vi "2 Cube Auto.vi"(11 "Right?":bool=TRUE) -> ()   [LabVIEW 2017]
uses:
  Auto Scale Type Def.ctl
  2 Cube Auto Type Def.ctl
  LabVIEW_is_Under_Control.lib/Util/Unpack Gamepad/D-Pad.ctl
  LabVIEW_is_Under_Control.lib/Util/Unpack Gamepad/Button Cluster.ctl
  Team Code/Robot Global Data.vi
panel:
  in  "String":string
  in  "DistanceFwd 4":dbl=600.0
  in  "Delay Fwd 4":i32=300
  in  "Time_Limit_fwd 4":dbl=5000.0 format="%#_13g"
  in  "Time_Limit_Turn 2":dbl=1000.0 format="%#_13g"
  in  "Turn 2":dbl=-30.0 format="%#_13g"
  in  "Delay Turn 2":i32=100
  in  "DistanceFwd 3":dbl=-60.0
  in  "Delay Fwd 3":i32=100
  in  "Time_Limit_fwd 3":dbl=1000.0 format="%#_13g"
  in  "Time to wait 3 (min 50ms)":dbl=100.0
  in  "DistanceFwd 2":dbl=55.0
  in  "Delay Fwd 2":i32=100
  in  "Time_Limit_fwd 2":dbl=1000.0 format="%#_13g"
  in  "Time to wait 2 (min 50ms)":dbl=100.0
  in  "Time_Limit_Turn":dbl=1000.0 format="%#_13g"
  in  "Turn":dbl=-30.0 format="%#_13g"
  in  "Delay Turn":i32=100
  in  "DistanceFwd":dbl=600.0
  in  "Delay Fwd":i32=300
  in  "Time_Limit_fwd":dbl=5000.0 format="%#_13g"
  in  "Time to wait (min 50ms)":dbl=100.0
  out "Auto state":T1=enum."Finalizando"
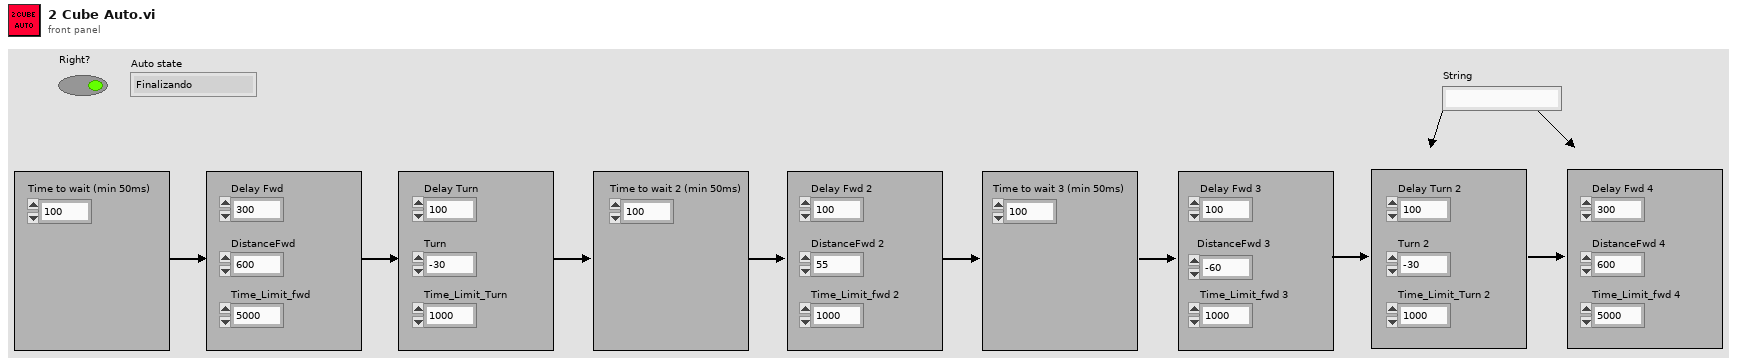
[diagram p1: front panel]
types:
  T1 = typedef "Auto Scale Type Def.ctl" = enum16{"Zerandosensor", "Andando", "Girando", "Zerandosensor2", "Andando2", "Score", "Zerandosensor3", "Andando3", "Finalizando"}
  T2 = typedef "2 Cube Auto Type Def.ctl" = enum16{"Zerandosensor", "Andando", "Girando", "Zerandosensor2", "Andando2", "Score", "Zerandosensor3", "Andando3", "Girando2", "Andando4", "Elevator Up", "Score2", "Finalizando"}
  T3 = typedef "D-Pad.ctl" = cluster{"Top":bool, "Bottom":bool, "None":bool, "Right":bool, "Left":bool}
  T4 = cluster{"proportional gain (Kc)":dbl, "integral time (Ti, min)":dbl, "derivative time (Td, min)":dbl}
  T5 = typedef "Button Cluster.ctl" = cluster{"Buttons[0]":bool, "Buttons[1]":bool, "Buttons[2]":bool, "Buttons[3]":bool, "Buttons[4]":bool, "Buttons[5]":bool, "Buttons[6]":bool, "Buttons[7]":bool, "Buttons[8]":bool, "Buttons[9]":bool}
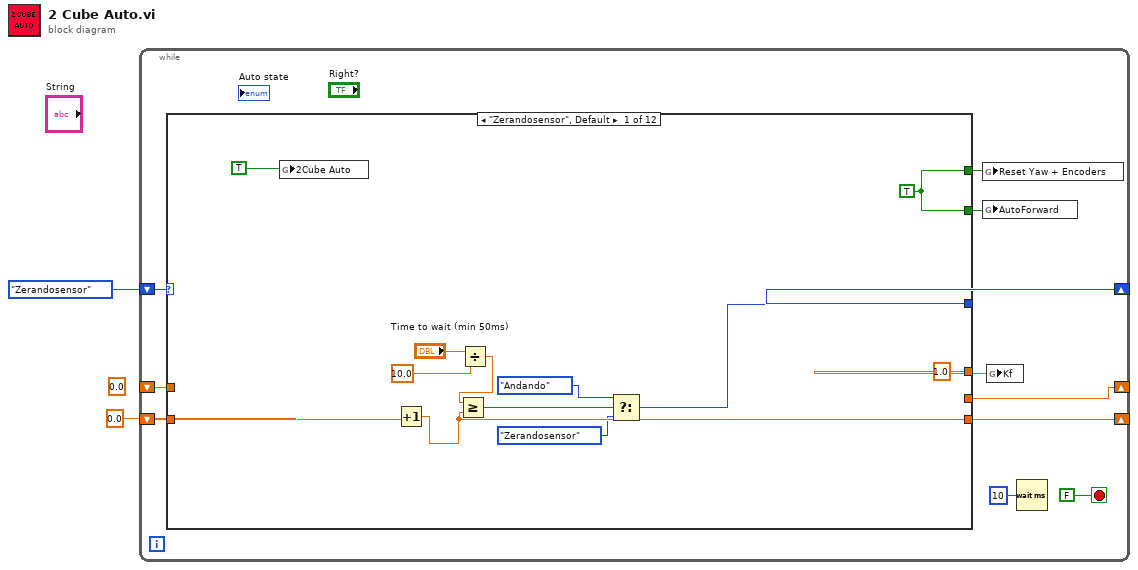
[diagram p0: block diagram]
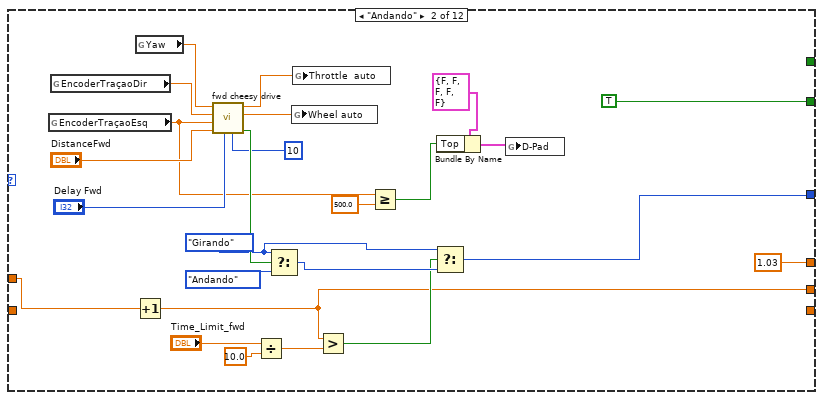
[diagram p2: hidden frame]
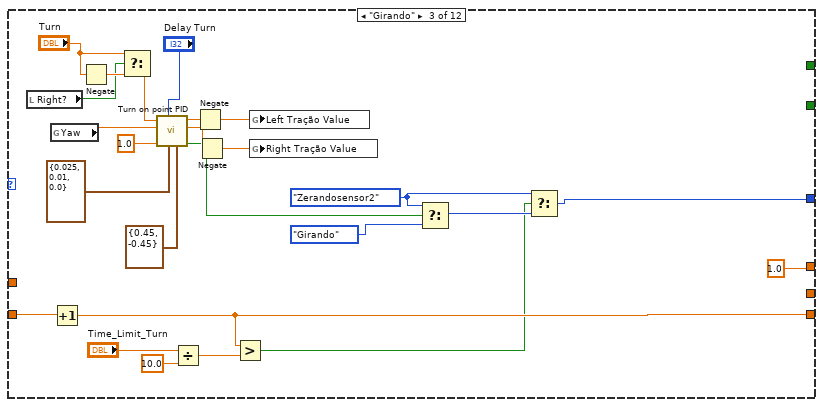
[diagram p3: hidden frame]
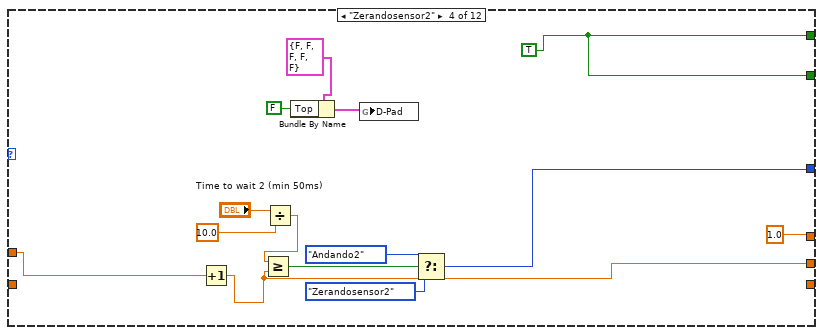
[diagram p4: hidden frame]
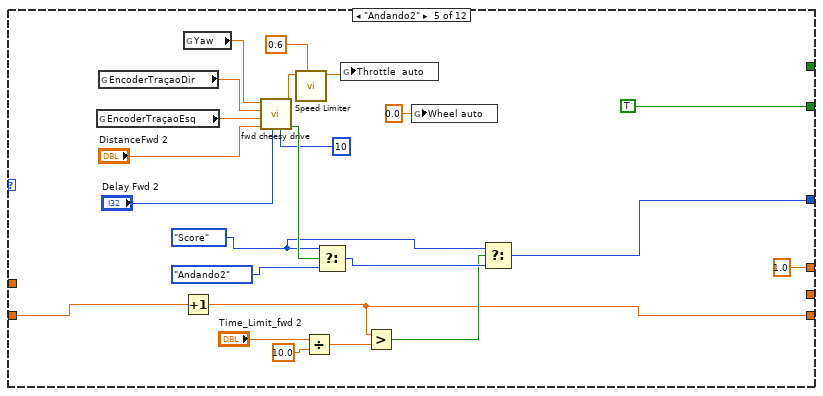
[diagram p5: hidden frame]
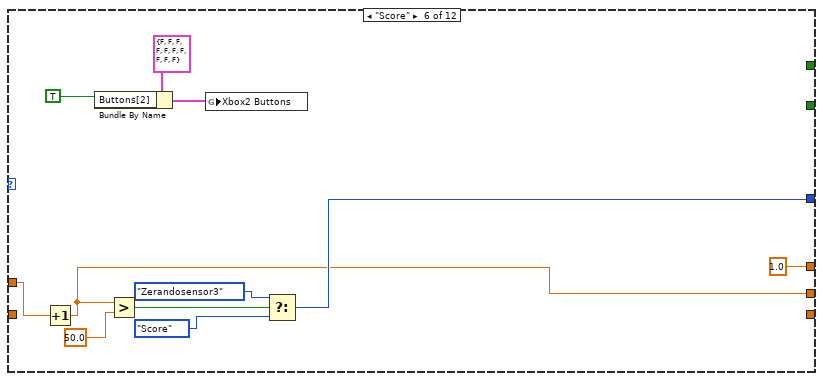
[diagram p6: hidden frame]
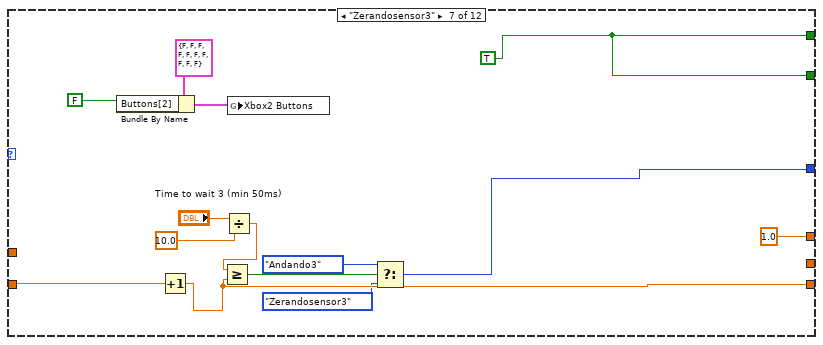
[diagram p7: hidden frame]
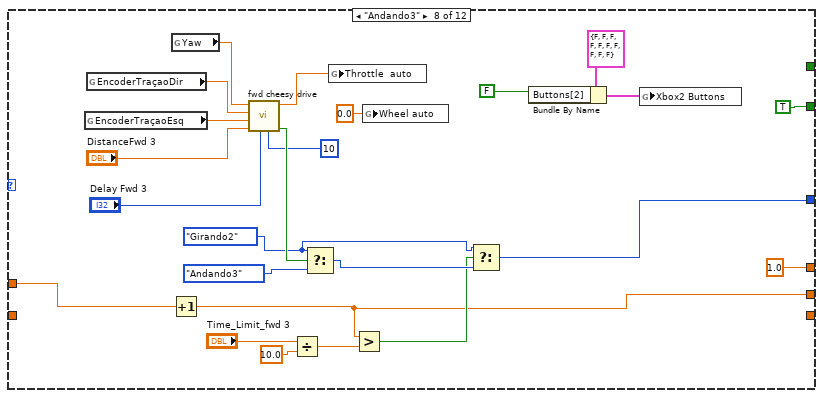
[diagram p8: hidden frame]
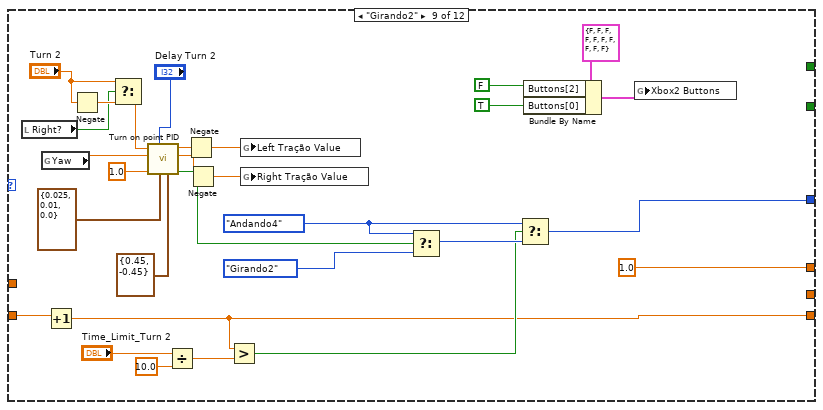
[diagram p9: hidden frame]
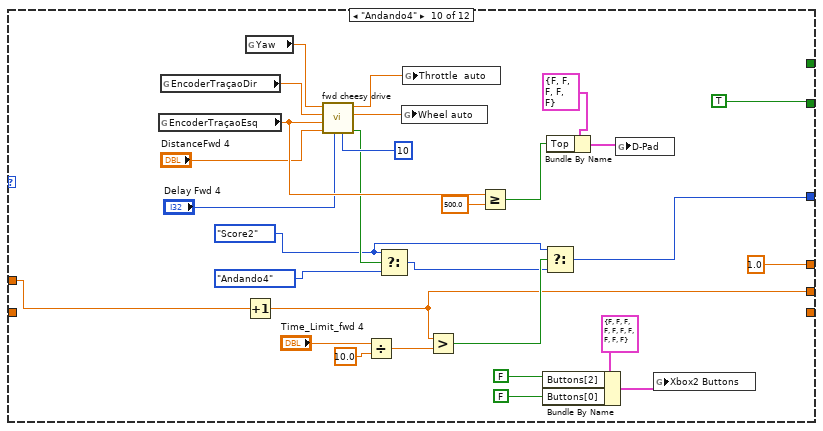
[diagram p10: hidden frame]
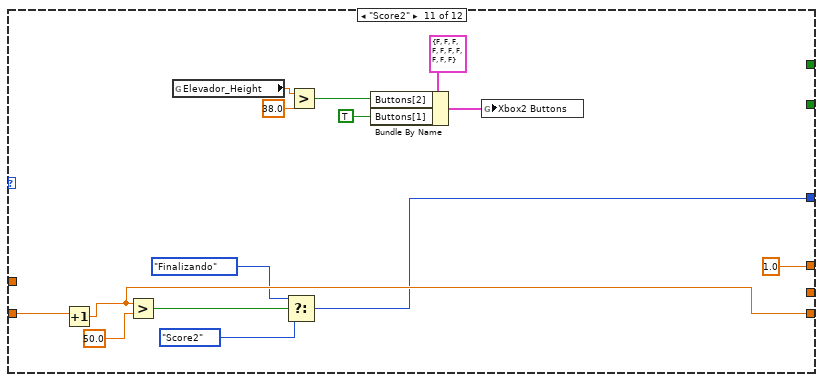
[diagram p11: hidden frame]
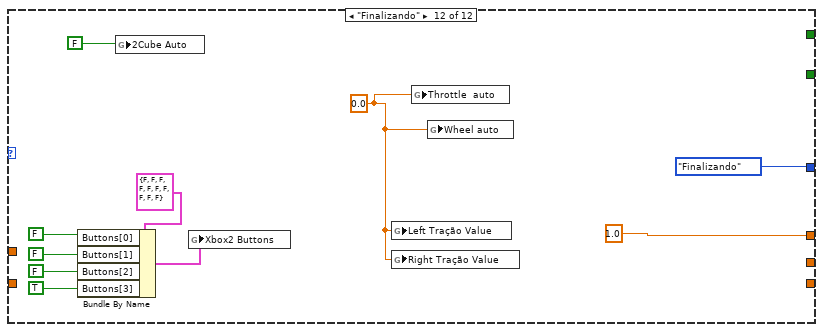
[diagram p12: hidden frame]
diagram:
  (unwired) 0.0
  n1 = while {
    shift-right: [w9] -> _
    shift-left: 2_Cube_Auto_Type_Def."Zerandosensor" ("Enum") -> [w3]
    shift-right: [w10] -> _
    shift-left: 0.0 -> [w11]
    shift-right: [w5] -> _
    shift-left: _ -> [w6]
    stop <- FALSE stop-if-true
    n2 = case shown="\"Zerandosensor\", Default" w3 {
      tunnel: w11 -> [w21 _ w72 _ w100 _ w131 _ w169 _ w228 _]
      tunnel: [w20 _ w71 _ w99 _ w130 _ w168 _ w227 _] -> w10
      tunnel: [w19 w43 w58 w83 w98 w118 w132 w146 w174 w195 w224 2_Cube_Auto_Type_Def."Finalizando" ("Enum")] -> w9
      tunnel: [w18 _ _ w82 _ _ w133 _ _ _ _ _] -> w8
      tunnel: [w18 TRUE _ w82 TRUE _ w133 TRUE _ TRUE _ _] -> w7
      tunnel: w6 -> [_ w36 _ w85 _ w117 _ w148 _ w200 _ _]
      tunnel: [_ w35 _ w84 _ w116 _ w147 _ w199 _ _] -> w5
      tunnel: [1.0 1.03 1.0 1.0 1.0 1.0 1.0 1.0 1.0 1.0 1.0 1.0] -> w4
      frame "Zerandosensor", Default {
        w18 = TRUE
        n3 = global write "Robot Global Data.vi" "2Cube Auto"(TRUE) -> ()
        n4 = Increment(x=w21) -> (x+1=w20:dbl)
        n5 = Divide(x="Time to wait (min 50ms)", y=10.0) -> (x/y=w23:dbl)
        n6 = Greater Or Equal?(x=w23, y=w20) -> (x >= y?=w22:bool)
        n7 = Select(t=2_Cube_Auto_Type_Def."Andando" ("Enum"), s=w22, f=2_Cube_Auto_Type_Def."Zerandosensor" ("Enum")) -> (s? t:f=w19:T2)
      }
      frame "Andando" {
        w27 = 2_Cube_Auto_Type_Def."Girando" ("Enum")
        n8 = global read "Robot Global Data.vi" "EncoderTraçaoEsq"() -> (w30:dbl)
        n9 = global read "Robot Global Data.vi" "EncoderTraçaoDir"() -> (w49:dbl)
        n10 = Increment(x=w36) -> (x+1=w35:dbl)
        n11 = global read "Robot Global Data.vi" "Yaw"() -> (w50:dbl)
        n12 = call "fwd cheesy drive.vi"("Loop Timer"=10, "Time to stop"="Delay Fwd", "Distance"="DistanceFwd", "Encoder Left"=w30, "Encoder Right"=w49, "Yaw"=w50) -> ("Finished distance"=w37:bool, "Direction"=w47:dbl, "Trottle"=w46:dbl)  [unwired: 2 in, 1 out]
        n13 = Divide(x="Time_Limit_fwd", y=10.0) -> (x/y=w42:dbl)
        n14 = Select(t=w27, s=w37, f=2_Cube_Auto_Type_Def."Andando" ("Enum")) -> (s? t:f=w44:T2)
        n15 = global write "Robot Global Data.vi" "Wheel auto"(w47) -> ()
        n16 = global write "Robot Global Data.vi" "Throttle  auto"(w46) -> ()
        n17 = Greater?(x=w35, y=w42) -> (0:w39:bool)
        n18 = Greater Or Equal?(x=w30, y=500.0) -> (x >= y?=w31:bool)
        n19 = Select(t=w27, s=w39, f=w44) -> (s? t:f=w43:T2)
        n20 = Bundle By Name(cluster=T3 {"Top"=FALSE, "Bottom"=FALSE, "None"=FALSE, "Right"=FALSE, "Left"=FALSE} ("D-Pad"), "Top"=w31) -> (w33:T3)
        n21 = global write "Robot Global Data.vi" "D-Pad"(w33) -> ()
      }
      frame "Girando" {
        w54 = 2_Cube_Auto_Type_Def."Zerandosensor2" ("Enum")
        n22 = local read "Right?"() -> (w51:bool)
        n23 = global read "Robot Global Data.vi" "Yaw"() -> (w67:dbl)
        n24 = Increment(x=w72) -> (x+1=w71:dbl)
        n25 = Negate(x="Turn") -> (-x=w57:dbl)
        n26 = Select(t="Turn", s=w51, f=w57) -> (s? t:f=w55:dbl)
        n27 = call "Turn on point PID.vi"("Range"=cluster{"output high":dbl, "output low":dbl} {"output high"=0.45, "output low"=-0.45}, "Gains"=T4 {"proportional gain (Kc)"=0.025, "integral time (Ti, min)"=0.01, "derivative time (Td, min)"=0.0}, "Time to stop"="Delay Turn", "Precision"=1.0, "Yaw"=w67, "Setpoint(degrees)"=w55) -> ("Finished?"=w63:bool, "PWM right"=w66:dbl, "PWM left"=w65:dbl)  [unwired: 3 in]
        n28 = Divide(x="Time_Limit_Turn", y=10.0) -> (x/y=w74:dbl)
        n29 = Negate(x=w65) -> (-x=w68:dbl)
        n30 = Negate(x=w66) -> (-x=w69:dbl)
        n31 = Greater?(x=w71, y=w74) -> (0:w59:bool)
        n32 = global write "Robot Global Data.vi" "Left Tração Value"(w68) -> ()
        n33 = global write "Robot Global Data.vi" "Right Tração Value"(w69) -> ()
        n34 = Select(t=w54, s=w63, f=2_Cube_Auto_Type_Def."Girando" ("Enum")) -> (s? t:f=w70:T2)
        n35 = Select(t=w54, s=w59, f=w70) -> (s? t:f=w58:T2)
      }
      frame "Zerandosensor2" {
        w82 = TRUE
        n36 = Increment(x=w85) -> (x+1=w84:dbl)
        n37 = Divide(x="Time to wait 2 (min 50ms)", y=10.0) -> (x/y=w87:dbl)
        n38 = Greater Or Equal?(x=w87, y=w84) -> (x >= y?=w86:bool)
        n39 = Bundle By Name(cluster=T3 {"Top"=FALSE, "Bottom"=FALSE, "None"=FALSE, "Right"=FALSE, "Left"=FALSE} ("D-Pad"), "Top"=FALSE) -> (w81:T3)
        n40 = global write "Robot Global Data.vi" "D-Pad"(w81) -> ()
        n41 = Select(t=2_Cube_Auto_Type_Def."Andando2" ("Enum"), s=w86, f=2_Cube_Auto_Type_Def."Zerandosensor2" ("Enum")) -> (s? t:f=w83:T2)
      }
      frame "Andando2" {
        w91 = 2_Cube_Auto_Type_Def."Score" ("Enum")
        n42 = global read "Robot Global Data.vi" "EncoderTraçaoEsq"() -> (w111:dbl)
        n43 = global read "Robot Global Data.vi" "EncoderTraçaoDir"() -> (w110:dbl)
        n44 = Increment(x=w100) -> (x+1=w99:dbl)
        n45 = global read "Robot Global Data.vi" "Yaw"() -> (w112:dbl)
        n46 = call "fwd cheesy drive.vi"("Loop Timer"=10, "Time to stop"="Delay Fwd 2", "Distance"="DistanceFwd 2", "Encoder Left"=w111, "Encoder Right"=w110, "Yaw"=w112) -> ("Finished distance"=w102:bool, "Trottle"=w94:dbl)  [unwired: 2 in, 2 out]
        n47 = call "Speed Limiter.vi"("Limit"=0.6, "Motor Input"=w94) -> ("Output"=w95:dbl)  [unwired: 9 in]
        n48 = Divide(x="Time_Limit_fwd 2", y=10.0) -> (x/y=w106:dbl)
        n49 = Select(t=w91, s=w102, f=2_Cube_Auto_Type_Def."Andando2" ("Enum")) -> (s? t:f=w107:T2)
        n50 = global write "Robot Global Data.vi" "Throttle  auto"(w95) -> ()
        n51 = Greater?(x=w99, y=w106) -> (0:w103:bool)
        n52 = global write "Robot Global Data.vi" "Wheel auto"(0.0 ("Wheel auto")) -> ()
        n53 = Select(t=w91, s=w103, f=w107) -> (s? t:f=w98:T2)
      }
      frame "Score" {
        n54 = Increment(x=w117) -> (x+1=w116:dbl)
        n55 = Bundle By Name(cluster=T5 {"Buttons[0]"=FALSE, "Buttons[1]"=FALSE, "Buttons[2]"=FALSE, "Buttons[3]"=FALSE, "Buttons[4]"=FALSE, "Buttons[5]"=FALSE, "Buttons[6]"=FALSE, "Buttons[7]"=FALSE, "Buttons[8]"=FALSE, "Buttons[9]"=FALSE} ("Xbox Buttons"), "Buttons[2]"=TRUE) -> (w122:T5)
        n56 = Greater?(x=w116, y=50.0) -> (0:w119:bool)
        n57 = global write "Robot Global Data.vi" "Xbox2 Buttons"(w122) -> ()
        n58 = Select(t=2_Cube_Auto_Type_Def."Zerandosensor3" ("Enum"), s=w119, f=2_Cube_Auto_Type_Def."Score" ("Enum")) -> (s? t:f=w118:T2)
      }
      frame "Zerandosensor3" {
        w133 = TRUE
        n59 = Bundle By Name(cluster=T5 {"Buttons[0]"=FALSE, "Buttons[1]"=FALSE, "Buttons[2]"=FALSE, "Buttons[3]"=FALSE, "Buttons[4]"=FALSE, "Buttons[5]"=FALSE, "Buttons[6]"=FALSE, "Buttons[7]"=FALSE, "Buttons[8]"=FALSE, "Buttons[9]"=FALSE} ("Xbox Buttons"), "Buttons[2]"=FALSE) -> (w125:T5)
        n60 = Increment(x=w131) -> (x+1=w130:dbl)
        n61 = Divide(x="Time to wait 3 (min 50ms)", y=10.0) -> (x/y=w135:dbl)
        n62 = Greater Or Equal?(x=w135, y=w130) -> (x >= y?=w134:bool)
        n63 = global write "Robot Global Data.vi" "Xbox2 Buttons"(w125) -> ()
        n64 = Select(t=2_Cube_Auto_Type_Def."Andando3" ("Enum"), s=w134, f=2_Cube_Auto_Type_Def."Zerandosensor3" ("Enum")) -> (s? t:f=w132:T2)
      }
      frame "Andando3" {
        w142 = 2_Cube_Auto_Type_Def."Girando2" ("Enum")
        n65 = global read "Robot Global Data.vi" "EncoderTraçaoEsq"() -> (w160:dbl)
        n66 = global read "Robot Global Data.vi" "EncoderTraçaoDir"() -> (w159:dbl)
        n67 = Increment(x=w148) -> (x+1=w147:dbl)
        n68 = global read "Robot Global Data.vi" "Yaw"() -> (w161:dbl)
        n69 = call "fwd cheesy drive.vi"("Loop Timer"=10, "Time to stop"="Delay Fwd 3", "Distance"="DistanceFwd 3", "Encoder Left"=w160, "Encoder Right"=w159, "Yaw"=w161) -> ("Finished distance"=w150:bool, "Trottle"=w157:dbl)  [unwired: 2 in, 2 out]
        n70 = Divide(x="Time_Limit_fwd 3", y=10.0) -> (x/y=w154:dbl)
        n71 = Select(t=w142, s=w150, f=2_Cube_Auto_Type_Def."Andando3" ("Enum")) -> (s? t:f=w155:T2)
        n72 = global write "Robot Global Data.vi" "Throttle  auto"(w157) -> ()
        n73 = Greater?(x=w147, y=w154) -> (0:w151:bool)
        n74 = global write "Robot Global Data.vi" "Wheel auto"(0.0 ("Wheel auto")) -> ()
        n75 = Select(t=w142, s=w151, f=w155) -> (s? t:f=w146:T2)
        n76 = Bundle By Name(cluster=T5 {"Buttons[0]"=FALSE, "Buttons[1]"=FALSE, "Buttons[2]"=FALSE, "Buttons[3]"=FALSE, "Buttons[4]"=FALSE, "Buttons[5]"=FALSE, "Buttons[6]"=FALSE, "Buttons[7]"=FALSE, "Buttons[8]"=FALSE, "Buttons[9]"=FALSE} ("Xbox Buttons"), "Buttons[2]"=FALSE) -> (w139:T5)
        n77 = global write "Robot Global Data.vi" "Xbox2 Buttons"(w139) -> ()
      }
      frame "Girando2" {
        w176 = 2_Cube_Auto_Type_Def."Andando4" ("Enum")
        n78 = local read "Right?"() -> (w166:bool)
        n79 = global read "Robot Global Data.vi" "Yaw"() -> (w180:dbl)
        n80 = Increment(x=w169) -> (x+1=w168:dbl)
        n81 = Negate(x="Turn 2") -> (-x=w188:dbl)
        n82 = Select(t="Turn 2", s=w166, f=w188) -> (s? t:f=w190:dbl)
        n83 = call "Turn on point PID.vi"("Range"=cluster{"output high":dbl, "output low":dbl} {"output high"=0.45, "output low"=-0.45}, "Gains"=T4 {"proportional gain (Kc)"=0.025, "integral time (Ti, min)"=0.01, "derivative time (Td, min)"=0.0}, "Time to stop"="Delay Turn 2", "Precision"=1.0, "Yaw"=w180, "Setpoint(degrees)"=w190) -> ("Finished?"=w184:bool, "PWM right"=w181:dbl, "PWM left"=w182:dbl)  [unwired: 3 in]
        n84 = Divide(x="Time_Limit_Turn 2", y=10.0) -> (x/y=w172:dbl)
        n85 = Negate(x=w182) -> (-x=w179:dbl)
        n86 = Negate(x=w181) -> (-x=w178:dbl)
        n87 = Greater?(x=w168, y=w172) -> (0:w170:bool)
        n88 = global write "Robot Global Data.vi" "Left Tração Value"(w179) -> ()
        n89 = global write "Robot Global Data.vi" "Right Tração Value"(w178) -> ()
        n90 = Select(t=w176, s=w184, f=2_Cube_Auto_Type_Def."Girando2" ("Enum")) -> (s? t:f=w177:T2)
        n91 = Select(t=w176, s=w170, f=w177) -> (s? t:f=w174:T2)
        n92 = Bundle By Name(cluster=T5 {"Buttons[0]"=FALSE, "Buttons[1]"=FALSE, "Buttons[2]"=FALSE, "Buttons[3]"=FALSE, "Buttons[4]"=FALSE, "Buttons[5]"=FALSE, "Buttons[6]"=FALSE, "Buttons[7]"=FALSE, "Buttons[8]"=FALSE, "Buttons[9]"=FALSE} ("Xbox Buttons"), "Buttons[2]"=FALSE, "Buttons[0]"=TRUE ("Buttons[1]")) -> (w164:T5)
        n93 = global write "Robot Global Data.vi" "Xbox2 Buttons"(w164) -> ()
      }
      frame "Andando4" {
        w196 = 2_Cube_Auto_Type_Def."Score2" ("Enum")
        n94 = global read "Robot Global Data.vi" "EncoderTraçaoEsq"() -> (w218:dbl)
        n95 = global read "Robot Global Data.vi" "EncoderTraçaoDir"() -> (w203:dbl)
        n96 = Increment(x=w200) -> (x+1=w199:dbl)
        n97 = global read "Robot Global Data.vi" "Yaw"() -> (w202:dbl)
        n98 = call "fwd cheesy drive.vi"("Loop Timer"=10, "Time to stop"="Delay Fwd 4", "Distance"="DistanceFwd 4", "Encoder Left"=w218, "Encoder Right"=w203, "Yaw"=w202) -> ("Finished distance"=w213:bool, "Direction"=w205:dbl, "Trottle"=w206:dbl)  [unwired: 2 in, 1 out]
        n99 = Divide(x="Time_Limit_fwd 4", y=10.0) -> (x/y=w209:dbl)
        n100 = Select(t=w196, s=w213, f=2_Cube_Auto_Type_Def."Andando4" ("Enum")) -> (s? t:f=w208:T2)
        n101 = global write "Robot Global Data.vi" "Wheel auto"(w205) -> ()
        n102 = global write "Robot Global Data.vi" "Throttle  auto"(w206) -> ()
        n103 = Greater?(x=w199, y=w209) -> (0:w212:bool)
        n104 = Greater Or Equal?(x=w218, y=500.0) -> (x >= y?=w217:bool)
        n105 = Bundle By Name(cluster=T5 {"Buttons[0]"=FALSE, "Buttons[1]"=FALSE, "Buttons[2]"=FALSE, "Buttons[3]"=FALSE, "Buttons[4]"=FALSE, "Buttons[5]"=FALSE, "Buttons[6]"=FALSE, "Buttons[7]"=FALSE, "Buttons[8]"=FALSE, "Buttons[9]"=FALSE} ("Xbox Buttons"), "Buttons[2]"=FALSE, "Buttons[0]"=FALSE ("Buttons[1]")) -> (w193:T5)
        n106 = Select(t=w196, s=w212, f=w208) -> (s? t:f=w195:T2)
        n107 = Bundle By Name(cluster=T3 {"Top"=FALSE, "Bottom"=FALSE, "None"=FALSE, "Right"=FALSE, "Left"=FALSE} ("D-Pad"), "Top"=w217) -> (w215:T3)
        n108 = global write "Robot Global Data.vi" "D-Pad"(w215) -> ()
        n109 = global write "Robot Global Data.vi" "Xbox2 Buttons"(w193) -> ()
      }
      frame "Score2" {
        n110 = Increment(x=w228) -> (x+1=w227:dbl)
        n111 = Greater?(x=w227, y=50.0) -> (0:w230:bool)
        n112 = global read "Robot Global Data.vi" "Elevador_Height"() -> (w222:dbl)
        n113 = Select(t=2_Cube_Auto_Type_Def."Finalizando" ("Enum"), s=w230, f=2_Cube_Auto_Type_Def."Score2" ("Enum")) -> (s? t:f=w224:T2)
        n114 = Greater?(x=w222, y=38.0) -> (0:w220:bool)
        n115 = Bundle By Name(cluster=T5 {"Buttons[0]"=FALSE, "Buttons[1]"=FALSE, "Buttons[2]"=FALSE, "Buttons[3]"=FALSE, "Buttons[4]"=FALSE, "Buttons[5]"=FALSE, "Buttons[6]"=FALSE, "Buttons[7]"=FALSE, "Buttons[8]"=FALSE, "Buttons[9]"=FALSE} ("Xbox Buttons"), "Buttons[2]"=w220, "Buttons[1]"=TRUE) -> (w233:T5)
        n116 = global write "Robot Global Data.vi" "Xbox2 Buttons"(w233) -> ()
      }
      frame "Finalizando" {
        w242 = 0.0
        n117 = Bundle By Name(cluster=T5 {"Buttons[0]"=FALSE, "Buttons[1]"=FALSE, "Buttons[2]"=FALSE, "Buttons[3]"=FALSE, "Buttons[4]"=FALSE, "Buttons[5]"=FALSE, "Buttons[6]"=FALSE, "Buttons[7]"=FALSE, "Buttons[8]"=FALSE, "Buttons[9]"=FALSE} ("Xbox Buttons"), "Buttons[0]"=FALSE ("Buttons[2]"), "Buttons[1]"=FALSE ("Buttons[3]"), "Buttons[2]"=FALSE ("Buttons[1]"), "Buttons[3]"=TRUE ("Buttons[0]")) -> (w243:T5)
        n118 = global write "Robot Global Data.vi" "2Cube Auto"(FALSE) -> ()
        n119 = global write "Robot Global Data.vi" "Xbox2 Buttons"(w243) -> ()
        n120 = global write "Robot Global Data.vi" "Left Tração Value"(w242) -> ()
        n121 = global write "Robot Global Data.vi" "Right Tração Value"(w242) -> ()
        n122 = global write "Robot Global Data.vi" "Throttle  auto"(w242) -> ()
        n123 = global write "Robot Global Data.vi" "Wheel auto"(w242) -> ()
      }
    }
    n124 = global write "Robot Global Data.vi" "Reset Yaw + Encoders"(w8) -> ()
    n125 = global write "Robot Global Data.vi" "AutoForward"(w7) -> ()
    n126 = global write "Robot Global Data.vi" "Kf"(w4) -> ()
    n127 = Wait (ms)(milliseconds to wait=u32 10) -> ()  [unwired: 1 out]
  }
